vi "Delete Header Content Line.vi"(8 "error in (no error)":errorcluster, 11 "Header in":refnum<class "Header.lvclass">) -> (0 "error out":errorcluster, 3 "Header out":refnum<class "Header.lvclass">)   [LabVIEW 2018]
uses:
  Header.lvclass
  C:/Users/observer/Desktop/SPARC4_ACS/Simulated_Header/Simulated_Header.lvclass
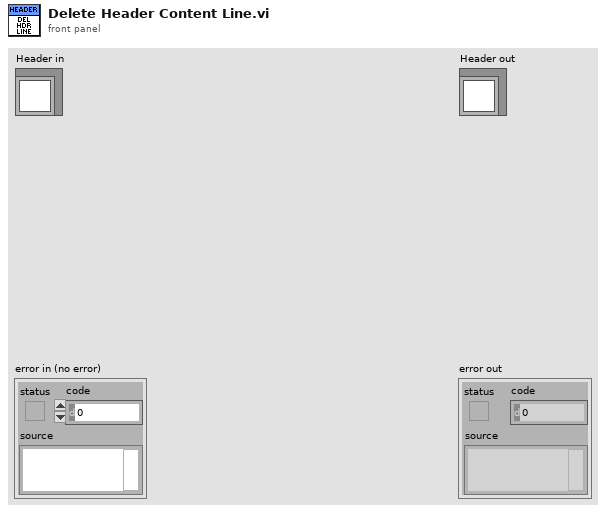
[diagram p1: front panel]
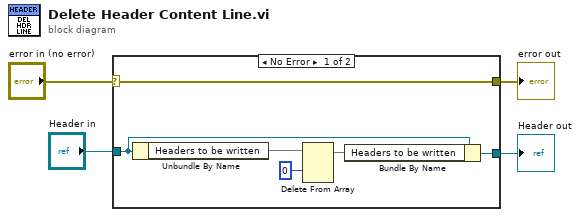
[diagram p0: block diagram]
diagram:
  n1 = case shown="No Error" "error in (no error)" {
    selector: "error in (no error)" -> [w10 w12]
    tunnel: [w10 w12] -> w3
    tunnel: [w6 w11] -> w1
    tunnel: "Header in" -> [w7 w11]
    frame No Error {
      n2 = Unbundle By Name(w7) -> ("Headers to be written"=w9)
      n3 = Delete From Array(array=w9, index (row)=0) -> (array with subset deleted=w5)  [unwired: 2 in, 1 out]
      n4 = Bundle By Name(cluster=w7, "Headers to be written"=w5) -> (w6:refnum<class "Header.lvclass">)
    }
    frame Error {
    }
  }
  "error out" <- w3
  "Header out" <- w1
